vi "serialRead_Write.vi"() -> ()   [LabVIEW 2019]
uses:
  Program Files/National Instruments/LabVIEW 2019/examples/Instrument IO/Serial/support/Serial - Settings.ctl
  <vilib>/Instr/_visa.llb/VISA Configure Serial Port (Instr).vi
  <vilib>/httpClient/POSTBuffer.vi
  <vilib>/httpClient/LabVIEWHTTPClient.lvlib
panel:
  out "Thermometer":dbl(slide) scale=0.0..100.0
  in  "VISA resource name":refnum<visa-resource-name>="COM1"
  in  "Stop":bool
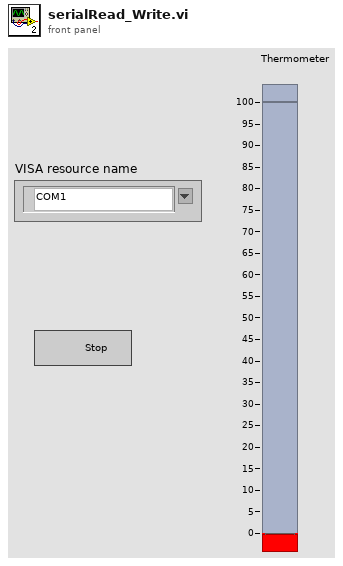
[diagram p1: front panel]
types:
  T1 = typedef "Serial - Settings.ctl" = cluster{"baud rate":u32, "data bits":u16, "parity":enum16{"None", "Odd", "Even", "Mark", "Space"}, "stop bits":u16, "flow control":u16}
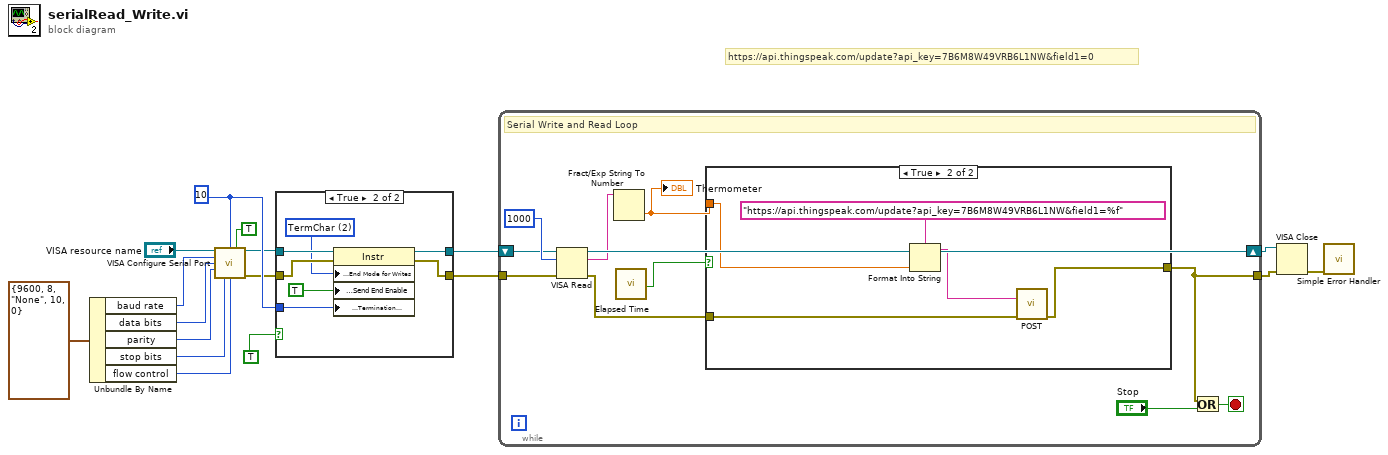
[diagram p0: block diagram]
diagram:
  w3 = u8 10 ("Termination Character")
  # "https://api.thingspeak.com/update?api_key=7B6M8W49VRB6L1NW&field1=0"
  n1 = Unbundle By Name(T1 {"baud rate"=9600, "data bits"=8, "parity"=enum."None", "stop bits"=10, "flow control"=0} ("Serial Settings")) -> ("baud rate"=w13:u32, "data bits"=w14:u16, "parity"=w15:enum16{"None", "Odd", "Even", "Mark", "Space"}, "stop bits"=w16:u16, "flow control"=w7:u16)
  n2 = call-poly "VISA Configure Serial Port"("VISA resource name"="VISA resource name", "termination char\n(0xA = '\\n' = LF)"=w3, "Enable Termination\nChar (T)"=TRUE ("End Read on Termination Character?"), "baud rate (9600)"=w13, "data bits (8)"=w14, "parity (0:none)"=w15, "stop bits (10: 1 bit)"=w16, "flow control (0:none)"=w7) -> ("VISA resource name out"=w2:refnum<visa-resource-name>, "error out"=w1:errorcluster)  [unwired: 2 in, 4 out]
  n3 = case shown="True" TRUE ("End Write on Termination Character?") {
    tunnel: w2 -> [w18 w26]
    tunnel: w1 -> [w19 w25]
    tunnel: [w18 w24] -> w5
    tunnel: [w19 w23] -> w6
    tunnel: w3 -> [_ w21]
    frame False {
    }
    frame True {
      w22 = u16 2 items=["None", "LastBit", "TermChar", "Break"] ("Serial Settings:Serial End Mode for Writes")
      n4 = property class="Instr"(reference=w26, error in=w25, "Serial Settings:End Mode for Writes"=w22, "Message Based Settings:Send End Enable"=TRUE, "Message Based Settings:Termination Character"=w21) -> (reference out=w24:refnum<visa-resource-name>, error out=w23:errorcluster)
    }
  }
  n5 = while {
    shift-right: [w37] -> w8
    shift-left: w5 -> [w33]
    tunnel: w6 -> [w32]
    tunnel: [w29] -> w9
    stop <- w36 stop-if-true
    # "Serial Write and Read Loop"
    n6 = VISA Read(VISA resource name=w33, byte count=u32 1000 ("Read Count"), error in (no error)=w32) -> (VISA resource name out=w37:refnum<visa-resource-name>, read buffer=w27:string, error out=w30:errorcluster)  [unwired: 1 out]
    n7 = Fract/Exp String To Number(string=w27) -> (number=w28:dbl)  [unwired: 3 in, 1 out]
    "Thermometer" <- w28
    n8 = call "Elapsed Time"() -> ("Time has Elapsed"=w31:bool)  [unwired: 12 in, 7 out]
    n9 = case shown="True" w31 {
      tunnel: w28 -> [_ w41]
      tunnel: [w38 w40] -> w29
      tunnel: w30 -> [w38 w39]
      frame False {
      }
      frame True {
        n10 = Format Into String(format string="https://api.thingspeak.com/update?api_key=7B6M8W49VRB6L1NW&field1=%f", w41) -> (resulting string=w43:string)  [unwired: 2 in, 1 out]
        n11 = call-poly <vilib>:"POST.vi"("url"=w43, "error in (no error)"=w39) -> ("error out"=w40:errorcluster)  [unwired: 10 in, 3 out]
      }
    }
    n12 = Or(x=w29, y="Stop") -> (x .or. y?=w36:bool)
  }
  n13 = VISA Close(VISA resource name=w8, error in (no error)=w9) -> (error out=w10:errorcluster)
  n14 = call <vilib>:"Simple Error Handler.vi"("error in (no error)"=w10) -> ()  [unwired: 1 in, 8 out]
